vi "Parse State Queue__jki_lib_state_machine.vi"(0 "State Queue":string, 7 "Error In (no error)":errorcluster) -> (4 "Remaining States":string, 6 "Current State":string, 8 "Arguments":string)   [LabVIEW 2013]
doc: "Parses the JKI State Machine state queue and returns the current state that will execute next with the associated arguments.\n\nFor instructions on how to use the JKI State Machine, examples and video tutorials, visit:\nhttp://jkisoft.com/state-machine/\n\n<B>Inputs:</B>\n <B>State Queue:</B> The entire state queue is wired to this input. This should come from the main JKI State Machine shift register.\n <B>Error In</B> The error cluster from the JKI State Machine is wired to this input. If an error occures and appears on this input, the current state output returns the \"Error Handler\" state.\n\n<B>Outputs:</B>\n <B>Remaining States:</B> Returns all the next states that should execute after the current state completes. These should be passed through the current state in the state machine. These can also be modified or augmented within the current state if necessary.\n <B>Current State:</B> Returns the current state that should execute next in the state machine. If an error is wired to the Error input then the current state output becomes \"Error Handler\".\n <B>Arguments:</B> Returns any argument(s) that may be used in the current state string. These arguments come after the \">>\" characters. <B>Note:</B> The arguments variable must not contain any unprintable characters like linefeed or carriage return.\n\n<B>State Syntax:</B>\nStateCategory: State >> Argument\nLine Terminator: Line feed\n <B>Example:</B>\nUI: Help >> About\n\nWhere \"UI\" is the state category\nWhere \"Help\" is the state\nWhere \"About\" is the argument\n <B>Other Examples:</B>\nApp Data: Initialize\nUI: Initialize\nHelp >> About\n\n<B>Commenting:</B>\nTo add a comment use \"//\" or \"#\" and all text to the right will be ignored\n <B>Commenting Example:</B>\nUI: Initialize // This initializes the UI\n# This whole line is a comment\n// Another comment line\n\nJKI State Machine™\nhttp://jkisoft.com/state-machine/\nCopyright (C) 2005-2008, JKI <info@jkisoft.com>\nALL RIGHTS RESERVED"
panel:
  # "For instructions on how to use the JKI State Machine, examples and video tutorials, visit:\nhttp://jkisoft.com/state-machine/\n\nJKI State Machine™\nhttp://jkisoft.com/state-machine/\nCopyright (C) 2005-2008, JKI <info@jkisoft.com>\nALL RIGHTS RESERVED"
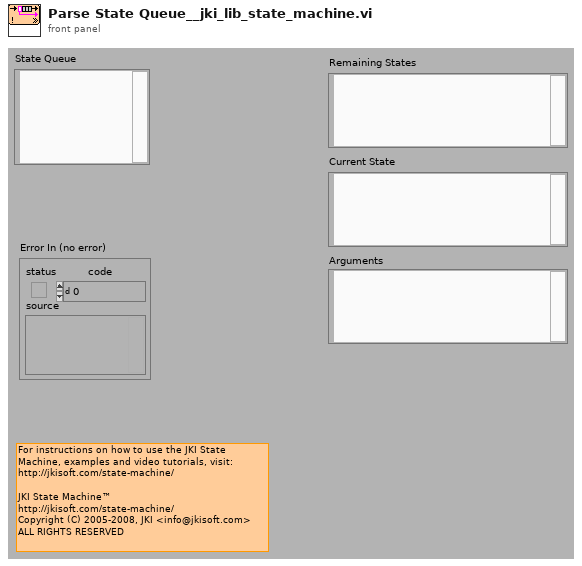
[diagram p1: front panel]
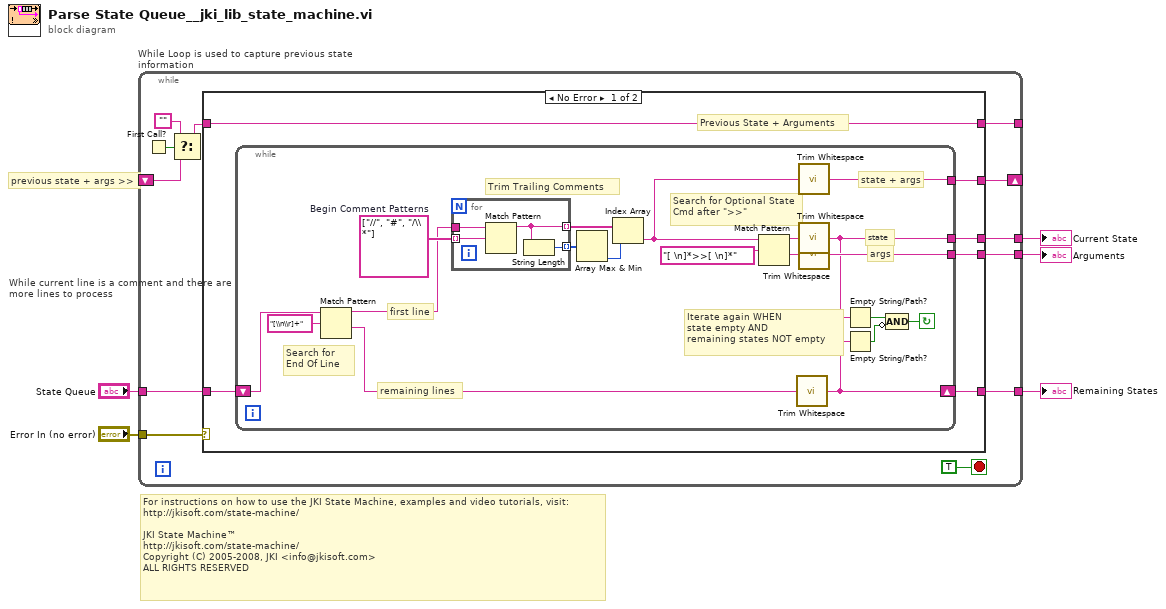
[diagram p0: block diagram]
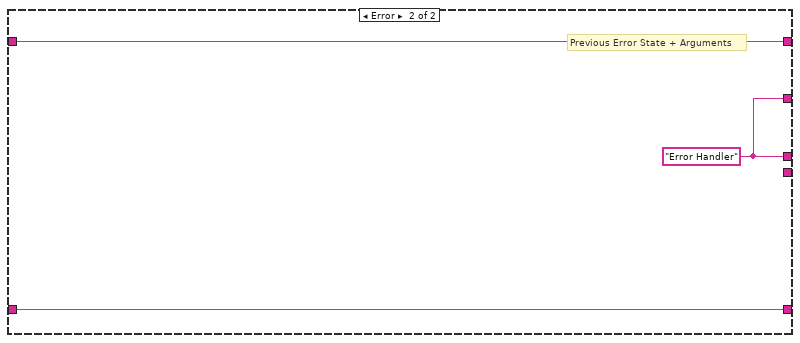
[diagram p2: hidden frame]
diagram:
  # "previous state + args >>"
  # "For instructions on how to use the JKI State Machine, examples and video tutorials, visit:\nhttp://jkisoft.com/state-machine/\n\nJKI State Machine™\nhttp://jkisoft.com/state-machine/\nCopyright (C) 2005-2008, JKI <info@jkisoft.com>\nALL RIGHTS RESERVED"
  n1 = while "While Loop is used to capture previous state information" {
    tunnel: [w17] -> w5
    tunnel: "State Queue" -> [w16]
    tunnel: "Error In (no error)" -> [w15]
    tunnel: [w14] -> w2
    tunnel: [w13] -> w1
    shift-right: [w11] -> _
    shift-left: _ -> [w9]
    tunnel: [w6] -> _
    stop <- TRUE stop-if-true
    n2 = First Call?() -> (First Call?: T/F=w10:bool)
    n3 = Select(t="", s=w10, f=w9) -> (s? t:f=w8:string)
    n4 = case shown="No Error" w15 {
      tunnel: [w20 w49] -> w17
      tunnel: [w23 w47] -> w14
      tunnel: [w22 _] -> w13
      tunnel: w16 -> [w21 w49]
      tunnel: [w19 w47] -> w11
      tunnel: w8 -> [w18 w48]
      tunnel: [w18 w48] -> w6
      frame No Error {
        # "Previous State + Arguments"
        n5 = while "While current line is a comment and there are more lines to process" {
          tunnel: [w33] -> w23
          tunnel: [w34] -> w22
          shift-right: [w29] -> w20
          shift-left: w21 -> [w27]
          tunnel: [w24] -> w19
          stop <- w30 continue-if-true
          w41 = string[] ["//", "#", "/\\*"]  # Begin Comment Patterns
          # "state + args"
          # "remaining lines"
          # "first line"
          # "Search for End Of Line"
          # "Iterate again WHEN\nstate empty AND\nremaining states NOT empty"
          # "args"
          # "state"
          # "Search for Optional State Cmd after \">>\""
          # "Trim Trailing Comments"
          n6 = Match Pattern(string=w27, regular expression="[\\n\\r]+") -> (before substring=w26:string, after substring=w42:string)  [unwired: 1 in, 2 out]
          n7 = for {
            tunnel: w26 -> [w46]
            tunnel: [w44] -> w38 mode=indexing
            tunnel: w41 -> [w45] mode=indexing
            tunnel: [w43] -> w40 mode=indexing
            n8 = Match Pattern(string=w46, regular expression=w45) -> (before substring=w44:string)  [unwired: 1 in, 3 out]
            n9 = String Length(string=w44) -> (length=w43:i32)
          }
          n10 = Array Max & Min(array=w40) -> (min index (indices)=w39:i32)  [unwired: 3 out]
          n11 = Index Array(array=w38, index=w39) -> (element=w25:string)
          n12 = Match Pattern(string=w25, regular expression="[ \n]*>>[ \n]*") -> (before substring=w36:string, after substring=w35:string)  [unwired: 1 in, 2 out]
          n13 = call "Trim Whitespace.vi"("string"=w42) -> ("trimmed string"=w29:string)  [unwired: 1 in]
          n14 = call "Trim Whitespace.vi"("string"=w25) -> ("trimmed string"=w24:string)  [unwired: 1 in]
          n15 = call "Trim Whitespace.vi"("string"=w36) -> ("trimmed string"=w33:string)  [unwired: 1 in]
          n16 = call "Trim Whitespace.vi"("string"=w35) -> ("trimmed string"=w34:string)  [unwired: 1 in]
          n17 = Empty String/Path?(string/path=w33) -> (empty?=w32:bool)
          n18 = Empty String/Path?(string/path=w29) -> (empty?=w31:bool)
          n19 = Compound Arithmetic op=AND(w32, invert w31) -> (w30:bool)
        }
      }
      frame Error {
        w47 = "Error Handler"
        # "Previous Error State + Arguments"
      }
    }
  }
  "Remaining States" <- w5
  "Arguments" <- w1
  "Current State" <- w2
